vi "Write CFG File.vi"(8 "error in (no error)":errorcluster, 10 "File path":path, 11 "Mag Lab Measure Controller in":refnum<class "Mag Lab Measure Controller.lvclass">) -> (0 "error out":errorcluster, 2 "Section":string, 3 "Mag Lab Measure Controller out":refnum<class "Mag Lab Measure Controller.lvclass">)   [LabVIEW 2015, in "Mag Lab Measure Controller.lvclass"]
uses:
  Mag Lab Measure Controller.lvclass
  Mag Lab Root Messages/Write CFG File Msg/Write CFG File Msg.lvclass/Write CFG File Msg.ctl
  <vilib>/ActorFramework/Message Enqueuer/Message Enqueuer.lvclass/Message Enqueuer.ctl
  <vilib>/ActorFramework/Message Enqueuer/Enqueue.vi
  <vilib>/ActorFramework/Message Priority Queue/Priority Enqueue.vi
  Compound Measurement/Compound Measurement.lvclass
  Mag Lab Root Messages/Write CFG File Msg/Write CFG File Msg.lvclass
  Mag Lab Measure Base/Mag Lab Measure Base.lvclass
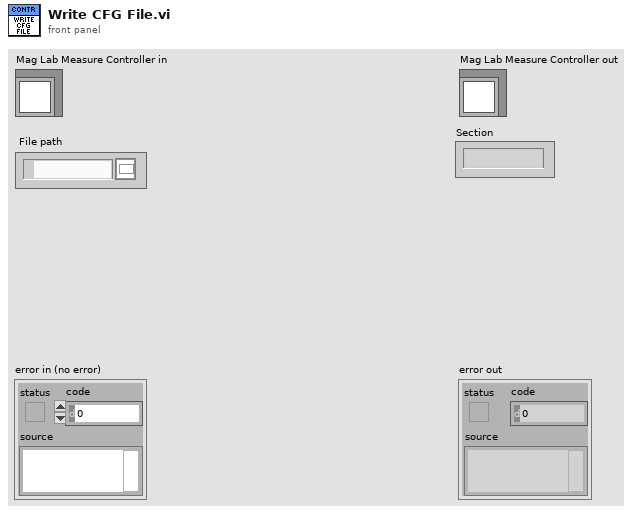
[diagram p1: front panel]
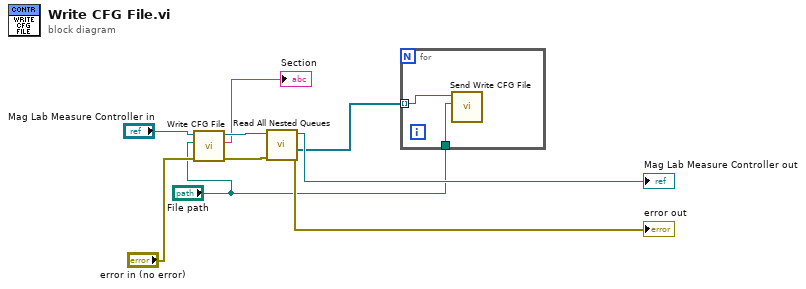
[diagram p0: block diagram]
diagram:
  n1 = call-parent "Write CFG File.vi"("error in (no error)"="error in (no error)", "File path"="File path", "Mag Lab Root in"="Mag Lab Measure Controller in") -> ("error out"=w4:errorcluster, "Section"=→"Section":string, "Mag Lab Root out"=w6:refnum<class "Mag Lab Measure Controller.lvclass">)  [unwired: 6 in]
  n2 = call "Read All Nested Queues.vi"("error in (no error)"=w4, "Mag Lab Measure Base in"=w6) -> ("error out"=→"error out":errorcluster, "Array of Queues"=w7:refnum<class "Message Enqueuer.lvclass">[], "Mag Lab Measure Base out"=→"Mag Lab Measure Controller out":refnum<class "Mag Lab Measure Controller.lvclass">)  [unwired: 6 in, 1 out]
  n3 = for {
    tunnel: w7 -> [w11] mode=indexing
    tunnel: "File path" -> [w10]
    n4 = call "Send Write CFG File.vi"("File path"=w10, "Message Enqueuer"=w11) -> ()  [unwired: 8 in, 2 out]
  }
